vi "test b-field creation.vi"() -> ()   [LabVIEW 2017]
uses:
  typedefs/magnet location fit result.ctl
  typedefs/magnetomter reading set.ctl
panel:
  out "size(s) 2":i32[](array[numeric])
  out "size(s)":i32
  out "derivative":dbl[][](array[numeric])
  in  "element":T1={"time"=240215635.0, "mag readings"=[{"magnetometer index"=0.0, "Bx"=-0.94140625, "By"=1.1923828125, "Bz"=-2.115234375, "magnetometer x"=0.0, "magnetometer y"=0.0}, {"magnetometer index"=0.0, "Bx"=-0.94140625, "By"=1.1923828125, "Bz"=-2.115234375, "magnetometer x"=0.0, "magnetometer y"=0.0}, {"magnetometer index"=1.0, "Bx"=-0.5595703125, "By"=0.1982421875, "Bz"=-1.1396484375, "magnetometer x"=-22.5, "magnetometer y"=38.971}, {"magnetometer index"=1.0, "Bx"=-0.5595703125, "By"=0.1982421875, "Bz"=-1.1396484375, "magnetometer x"=-22.5, "magnetometer y"=38.971}, {"magnetometer index"=2.0, "Bx"=-0.2822265625, "By"=0.599609375, "Bz"=-1.201171875, "magnetometer x"=-22.5, "magnetometer y"=-38.971}, {"magnetometer index"=3.0, "Bx"=-0.6376953125, "By"=0.4404296875, "Bz"=-1.11328125, "magnetometer x"=45.0, "magnetometer y"=0.0}, {"magnetometer index"=2.0, "Bx"=-0.2822265625, "By"=0.599609375, "Bz"=-1.201171875, "magnetometer x"=-22.5, "magnetometer y"=-38.971}, {"magnetometer index"=3.0, "Bx"=-0.6376953125, "By"=0.4404296875, "Bz"=-1.11328125, "magnetometer x"=45.0, "magnetometer y"=0.0}]}
  out "measured field":dbl[][](array[numeric])
  out "predicted field":dbl[][](array[numeric])
  in  "magnet location params":T2={"x magnet"=0.0, "y magnet"=0.0, "z magnet"=75.0, "Br*V (T*mm^3)"=500.0, "theta - moment angle to z-axis"=0.0, "phi - moment angle to x-axis"=0.0}
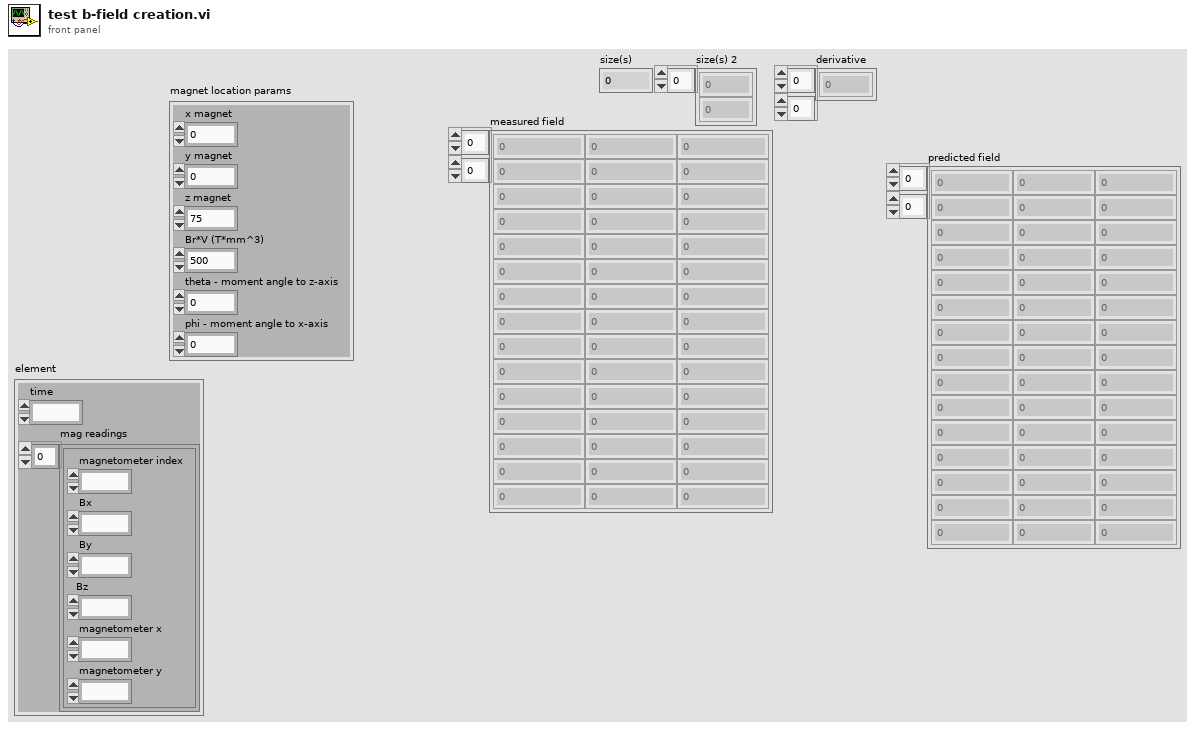
[diagram p1: front panel]
types:
  T1 = typedef "magnetomter reading set.ctl" = cluster{"time":fxp<+,48,48>, "mag readings":cluster{"magnetometer index":dbl, "Bx":dbl, "By":dbl, "Bz":dbl, "magnetometer x":dbl, "magnetometer y":dbl}[]}
  T2 = typedef "magnet location fit result.ctl" = cluster{"x magnet":dbl, "y magnet":dbl, "z magnet":dbl, "Br*V (T*mm^3)":dbl, "theta - moment angle to z-axis":dbl, "phi - moment angle to x-axis":dbl}
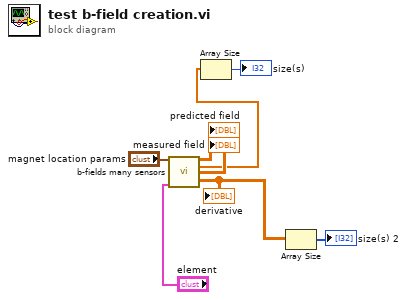
[diagram p0: block diagram]
diagram:
  n1 = call "b-fields many sensors.vi"("magnet location params"="magnet location params", "Magnetometer reading set"="element") -> ("predicted field"=→"predicted field":dbl[][], "pf - flat"=w4:dbl[], "measured field"=→"measured field":dbl[][], "derivative"=w2:dbl[][])  [unwired: 7 in, 3 out]
  "derivative" <- w2
  n2 = Array Size(array=w4) -> (size(s)=→"size(s)":i32)
  n3 = Array Size(array=w2) -> (size(s)=→"size(s) 2":i32[])
